vi "Write File.vi"(8 "Error In":errorcluster, 10 "File":path=path "", 11 "Known Hosts In":refnum<class "Known Hosts.lvclass">) -> (0 "Error Out":errorcluster, 3 "Known Hosts Out":refnum<class "Known Hosts.lvclass">)   [LabVIEW 2021, in "Field_RnD_Services_LIBSSH2_Toolkit.lvlib" / "Known Hosts.lvclass"]
doc: "Writes the current list of known hosts to a local file."
uses:
  Known Hosts.lvclass
  Known Hosts.lvclass/Known Hosts.ctl
  Field_RnD_Services_LIBSSH2_Toolkit.lvlib
  Session/Session.lvclass
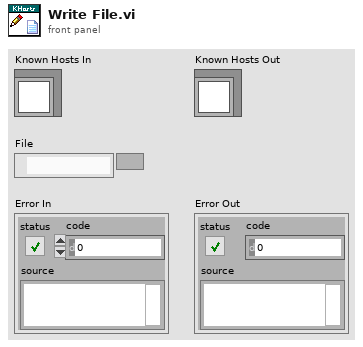
[diagram p1: front panel]
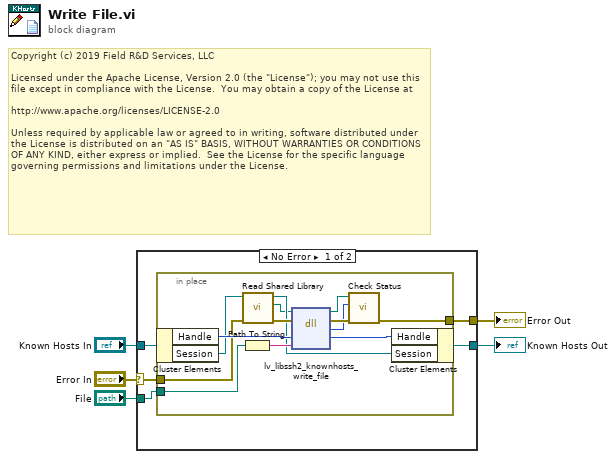
[diagram p0: block diagram]
diagram:
  # "Copyright (c) 2019 Field R&D Services, LLC\n\nLicensed under the Apache License, Version 2.0 (the \"License\"); you may not use this file except in compliance with the License.  You may obtain a copy of the License at\n\nhttp://www.apache.org/licenses/LICENSE-2.0\n\nUnless required by applicable law or agreed to in writing, software distributed under the License is distributed on an \"AS IS\" BASIS, WITHOUT WARRANTIES OR CONDITIONS OF ANY KIND, either express or implied.  See the License for the specific language governing permissions and limitations under the License."
  n1 = case shown="No Error" "Error In" {
    selector: "Error In" -> [w8 w25]
    tunnel: "Known Hosts In" -> [w10 w24]
    tunnel: [w7 w25] -> w3
    tunnel: [w9 w24] -> w2
    tunnel: "File" -> [w6 _]
    frame No Error {
      n2 = in-place {
        in-place-border: w8 -> [w16]
        in-place-border: [w19] -> w7
        in-place-border: w6 -> [w15]
        n3 = in-place-cluster #1(w10) -> ("Handle"=w23:u64, "Session"=w13:refnum<class "Session.lvclass">)
        n4 = Path To String(path=w15) -> (string=w17:string)
        n5 = call "Read Shared Library.vi"("Error In"=w16, "Session In"=w13) -> ("Erorr Out"=w14:errorcluster, "libssh2lv Shared Library"=w11:path, "Session Out"=w12:refnum<class "Session.lvclass">)  [unwired: 7 in]
        n6 = dll-call lib="D:/Users/cfield/Code/Field R&D Services/SSH/LV-LIBSSH2/LabVIEW/trunk/src/Toolkit/Support/lv-libssh2.*" fn="lv_libssh2_knownhosts_write_file"(path in=w11, error in=w14, "handle"=w23, "file"=w17) -> (path out=w20:path, error out=w21:errorcluster, "status"=w18:i32, "handle"=w22:u64)  [unwired: 2 in]
        n7 = call "Check Status.vi"("Error In"=w21, "Status"=w18, "libssh2lv Shared Library In"=w20) -> ("Error Out"=w19:errorcluster)  [unwired: 7 in, 1 out]
        n8 = in-place-cluster #1("Handle"=w22, "Session"=w12) -> (w9:refnum<class "Known Hosts.lvclass">)
      }
    }
    frame Error {
    }
  }
  "Error Out" <- w3
  "Known Hosts Out" <- w2
